vi "ts_tree_set_child.vi"(4 "results.data":string, 6 "results.txt":string, 8 "error in (no error)":errorcluster, 9 "ts.status":bool, 10 "ts.data":T1, 11 "Tree.in":refnum<vi>) -> (0 "error out":errorcluster, 3 "Tree.out":refnum<vi>)   [LabVIEW 2015]
doc: "sets a child test step results against the current active parent tag"
uses:
  ts-data.ctl
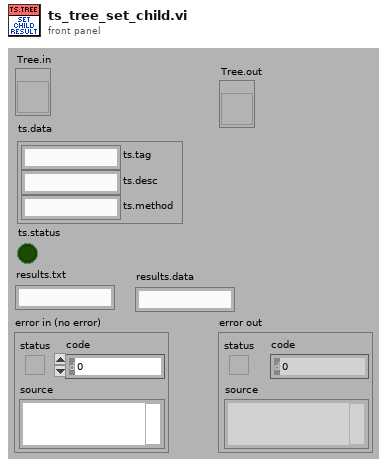
[diagram p1: front panel]
types:
  T1 = typedef "ts-data.ctl" = cluster{"ts.tag":string, "ts.desc":string, "ts.method":string}
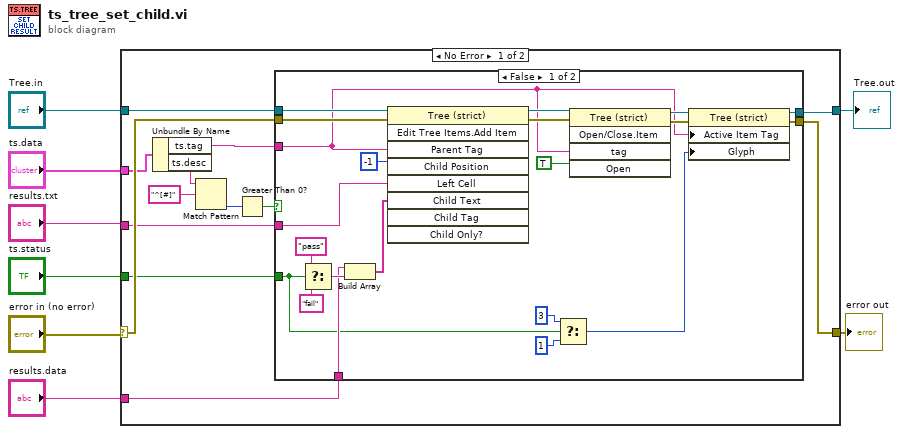
[diagram p0: block diagram]
diagram:
  n1 = case shown="No Error" "error in (no error)" {
    selector: "error in (no error)" -> [w21 w45]
    tunnel: "Tree.in" -> [w20 w46]
    tunnel: [w16 w46] -> w6
    tunnel: [w14 w45] -> w5
    tunnel: "ts.status" -> [w13 _]
    tunnel: "results.txt" -> [w19 _]
    tunnel: "ts.data" -> [w18 _]
    tunnel: "results.data" -> [w17 _]
    frame No Error {
      n2 = Unbundle By Name(w18) -> ("ts.tag"=w15:string, "ts.desc"=w9:string)
      n3 = Match Pattern(string=w9, regular expression="^[#]") -> (offset past match=w12:i32)  [unwired: 1 in, 3 out]
      n4 = Greater Than 0?(x=w12) -> (x > 0?=w10:bool)
      n5 = case shown="False" w10 {
        tunnel: w21 -> [w41 w44]
        tunnel: w20 -> [w39 w43]
        tunnel: w19 -> [w35 _]
        tunnel: w17 -> [w31 _]
        tunnel: [w28 w43] -> w16
        tunnel: w15 -> [w27 _]
        tunnel: [w26 w44] -> w14
        tunnel: w13 -> [w25 _]
        frame False {
          n6 = Select(t="pass", s=w25, f="fail") -> (s? t:f=w32:string)
          n7 = Build Array(w31, w32) -> (w30:string[])
          n8 = invoke class="Tree (strict)" method="Edit Tree Items.Add Item"(reference=w39, error in=w41, "Parent Tag"=w27, "Child Position"=-1, "Left Cell"=w35, "Child Text"=w30) -> (reference out=w37:refnum<vi>, error out=w36:errorcluster)  [unwired: 3 in, 7 out]
          n9 = Select(t=3, s=w25, f=1) -> (s? t:f=w22:i32)
          n10 = invoke class="Tree (strict)" method="Open/Close.Item"(reference=w37, error in=w36, "tag"=w27, "Open"=TRUE ("Open?")) -> (reference out=w29:refnum<vi>, error out=w42:errorcluster)  [unwired: 1 in, 3 out]
          n11 = property class="Tree (strict)"(reference=w29, error in=w42, "Active Item Tag"=w27, "Glyph"=w22) -> (reference out=w28:refnum<vi>, error out=w26:errorcluster)
        }
        frame True {
        }
      }
    }
    frame Error {
    }
  }
  "Tree.out" <- w6
  "error out" <- w5
